vi "prueba2_520.vi"() -> ()   [LabVIEW 2011]
panel:
  out "MayorTemp":dbl
  out "TEmp>40":bool
  out "contarTem>40":dbl
  out "promedioTempPares":dbl
  out "Thermometer":i32(slide) scale=0.0..60.0
  # "Deberá de generar 10 temperaturas  y contar cuantas \nson mayorea a 40,obtener el mayor de todas las temperatutas\n, el promedio de las temp pares."
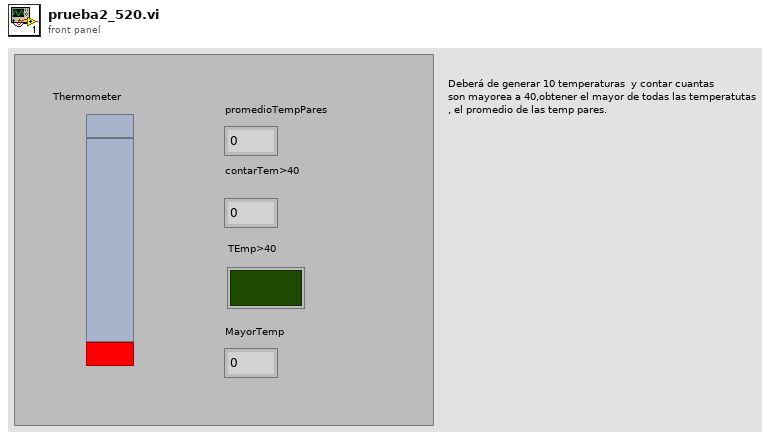
[diagram p1: front panel]
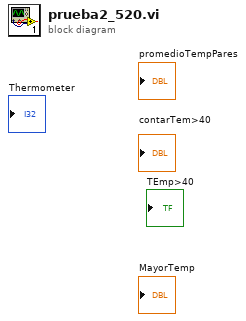
[diagram p0: block diagram]
diagram:
